vi "Get Target Specific Data.vi"(8 "error in (no error)":errorcluster, 11 "Operating System":string) -> (0 "error out":errorcluster, 2 "Skip?":bool, 3 "Target Specific Data":T1)   [LabVIEW 2014]
doc: "Gets the paths and settings specific to the specified OS"
uses:
  Target Specific Data.ctl
  Target Data Global.vi
  <vilib>/Utility/error.llb/Error Cluster From Error Code.vi
  <vilib>/ErrorRing/Error Ring.xnode
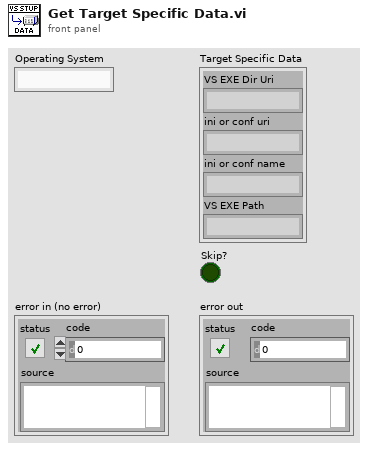
[diagram p1: front panel]
types:
  T1 = typedef "Target Specific Data.ctl" = cluster{"VS EXE Dir Uri":string, "ini or conf uri":string, "ini or conf name":string, "VS EXE Path":string}
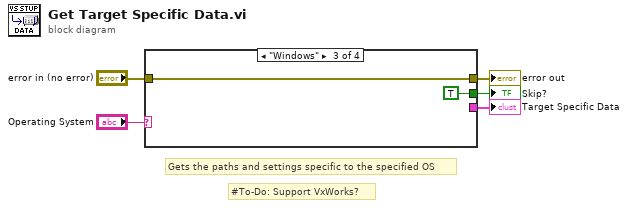
[diagram p0: block diagram]
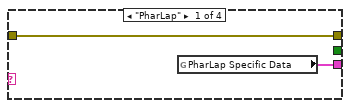
[diagram p2: hidden frame]
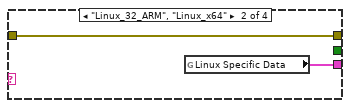
[diagram p3: hidden frame]
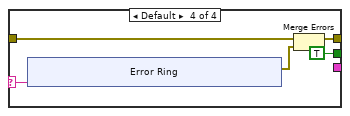
[diagram p4: hidden frame]
diagram:
  # "#To-Do: Support VxWorks?"
  # "Gets the paths and settings specific to the specified OS"
  n1 = case shown="\"Windows\"" "Operating System" {
    selector: "Operating System" -> [_ _ _ w16]
    tunnel: "error in (no error)" -> [w7 w9 w11 w14]
    tunnel: [w7 w9 w11 w13] -> w4
    tunnel: [w6 w8 _ _] -> w5
    tunnel: [_ _ TRUE TRUE] -> w1
    frame "PharLap" {
      n2 = global read "Target Data Global.vi" "PharLap Specific Data"() -> (w6:T1)
    }
    frame "Linux_32_ARM", "Linux_x64" {
      n3 = global read "Target Data Global.vi" "Linux Specific Data"() -> (w8:T1)
    }
    frame "Windows" {
    }
    frame Default {
      n4 = xnode "Error Ring"("parameter 0"=w16) -> ("error out"=w15:errorcluster)
      n5 = Merge Errors(w14, w15) -> (w13:errorcluster)
    }
  }
  "Target Specific Data" <- w5
  "error out" <- w4
  "Skip?" <- w1
